vi "G# - Property Example LV2010.vi"() -> ()   [LabVIEW 2017]
doc: "Property\nThis example shows how properties are used in LV2010, by using the property definition."
uses:
  MyPropertyClass_LV2010_class/MyPropertyClass_LV2010.lvclass
  <vilib>/addons/_AddQ/G#Object/G#Object.lvclass
panel:
  out "Name out":string
  in  "error in (no error)":errorcluster
  out "error out":errorcluster
  in  "Name":string="AddQ"
  # "Property\nThis example shows how properties are used in LV2010, by using the property definition."
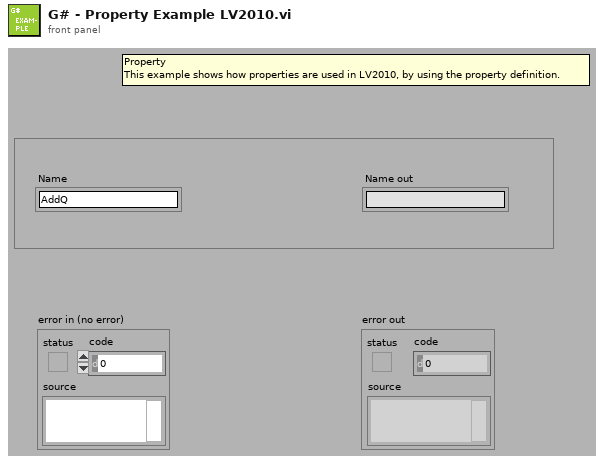
[diagram p1: front panel]
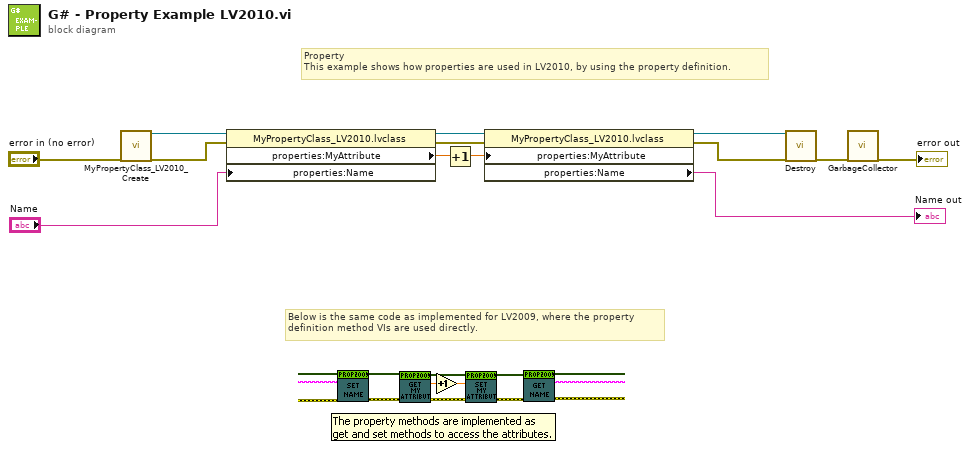
[diagram p0: block diagram]
diagram:
  # "Below is the same code as implemented for LV2009, where the property\ndefinition method VIs are used directly."
  # "Property\nThis example shows how properties are used in LV2010, by using the property definition."
  n1 = call "MyPropertyClass_LV2010_Create.vi"("error in (no error)"="error in (no error)") -> ("reference out"=w10:refnum<class "MyPropertyClass_LV2010.lvclass">, "error out"=w9:errorcluster)  [unwired: 17 in]
  n2 = property class="MyPropertyClass_LV2010.lvclass"(reference=w10, error in=w9, "properties:Name"="Name") -> (reference out=w6:refnum<class "MyPropertyClass_LV2010.lvclass">, error out=w7:errorcluster, "properties:MyAttribute"=w5:dbl)
  n3 = Increment(x=w5) -> (x+1=w4:dbl)
  n4 = property class="MyPropertyClass_LV2010.lvclass"(reference=w6, error in=w7, "properties:MyAttribute"=w4) -> (reference out=w2:refnum<class "MyPropertyClass_LV2010.lvclass">, error out=w3:errorcluster, "properties:Name"=→"Name out":string)
  n5 = call-dynamic "Destroy.vi"("reference in"=w2, "error in (no error)"=w3) -> ("error out"=w12:errorcluster)  [unwired: 16 in, 1 out]
  n6 = call <vilib>:"GarbageCollector.vi"("error in (no error)"=w12) -> ("error out"=→"error out":errorcluster)  [unwired: 16 in, 2 out]
